vi "Actor Core.vi"(8 "error in":errorcluster, 11 "PLC_Module in":refnum<class "PLC_Module.lvclass">) -> (0 "error out":errorcluster, 3 "Actor out":refnum<class "Actor.lvclass">)   [LabVIEW 2025, in "PLC_Module.lvlib" / "PLC_Module.lvclass"]
doc: "<p>(<strong>Filename</strong>: <span class=\"dnl\">Actor Framework.lvlib:Actor.lvclass:Actor Core.vi</span>)</p>\n<p>Receives messages to the actor, reacts to them, and initiates any error handling that may shut the actor down.</p>\n<p>Descendant classes may override this VI to append parallel tasks for the actor to complete while it handles messages. Overrides use the <a href=\"nihelplauncher://docs/csh?context=lvcore_glang_udclass\">Call Parent Class Method</a> node.</p>"
uses:
  PLC_Module.lvclass
  <vilib>/ActorFramework/Actor/Actor.lvclass
  Msg&Data.ctl
  Msg.ctl
  PLC_Module.lvclass/PLC_Module.ctl
  <vilib>/ActorFramework/Actor/Actor.lvclass/Actor.ctl
  <vilib>/ActorFramework/Message Enqueuer/Message Enqueuer.lvclass/Message Enqueuer.ctl
  PLC_Module Messages/Rename Msg/Rename Msg.lvclass/Rename Msg.ctl
  PLC_Module Messages/Set Data Msg/Set Data Msg.lvclass/Set Data Msg.ctl
  PLC_Module Messages/Write Monitor Msg/Write Monitor Msg.lvclass/Write Monitor Msg.ctl
  UI_Object.ctl
  PLC_Module Messages/UI_Initialize Msg/UI_Initialize Msg.lvclass/UI_Initialize Msg.ctl
  PLC_Module Messages/Connection Msg/Connection Msg.lvclass/Connection Msg.ctl
  PLC_Module Messages/EditPanel Msg/EditPanel Msg.lvclass/EditPanel Msg.ctl
  <vilib>/addons/_JKI Toolkits/State Machine/_JKI_lib_State_Machine.llb/Select State(s)_err__jki_lib_state_machine.vi
  Read Configuration.vi
  Read ModuleName.vi
  Read ConnectConfig.vi
  Write ConnectConfig.vi
  <vilib>/ActorFramework/Message Enqueuer/Init from Existing Queue.vi
  <vilib>/ActorFramework/Message Enqueuer/Enqueue.vi
  PLC_Module Messages/PanelClose Msg/PanelClose Msg.lvclass
  PLC_Module Messages/Rename Msg/Rename Msg.lvclass
  PLC_Module Messages/Set Data Msg/Set Data Msg.lvclass
  PLC_Module Messages/Write Monitor Msg/Write Monitor Msg.lvclass
  <vilib>/ActorFramework/Stop Msg/Stop Msg.lvclass
  PLC_Module Messages/UI_Initialize Msg/UI_Initialize Msg.lvclass
  PLC_Module Messages/Monitor Msg/Monitor Msg.lvclass
  PLC_Module Messages/Connection Msg/Connection Msg.lvclass
  PLC_Module Messages/Disconnection Msg/Disconnection Msg.lvclass
  PLC_Module Messages/EditPanel Msg/EditPanel Msg.lvclass
  PLC_Module Messages/Delete Item Msg/Delete Item Msg.lvclass
  PLC_Module Messages/DuplicateItem Msg/DuplicateItem Msg.lvclass
  <vilib>/addons/_JKI Toolkits/State Machine/_JKI_lib_State_Machine.llb/Periodic Trigger__ogtk__JKI-SM__jki_lib_state_machine.vi
  <vilib>/ActorFramework/Message Priority Queue/Priority Enqueue.vi
  <vilib>/ActorFramework/Message Enqueuer/Message Enqueuer.lvclass
panel:
  in  "Listbox":i32[](listbox)
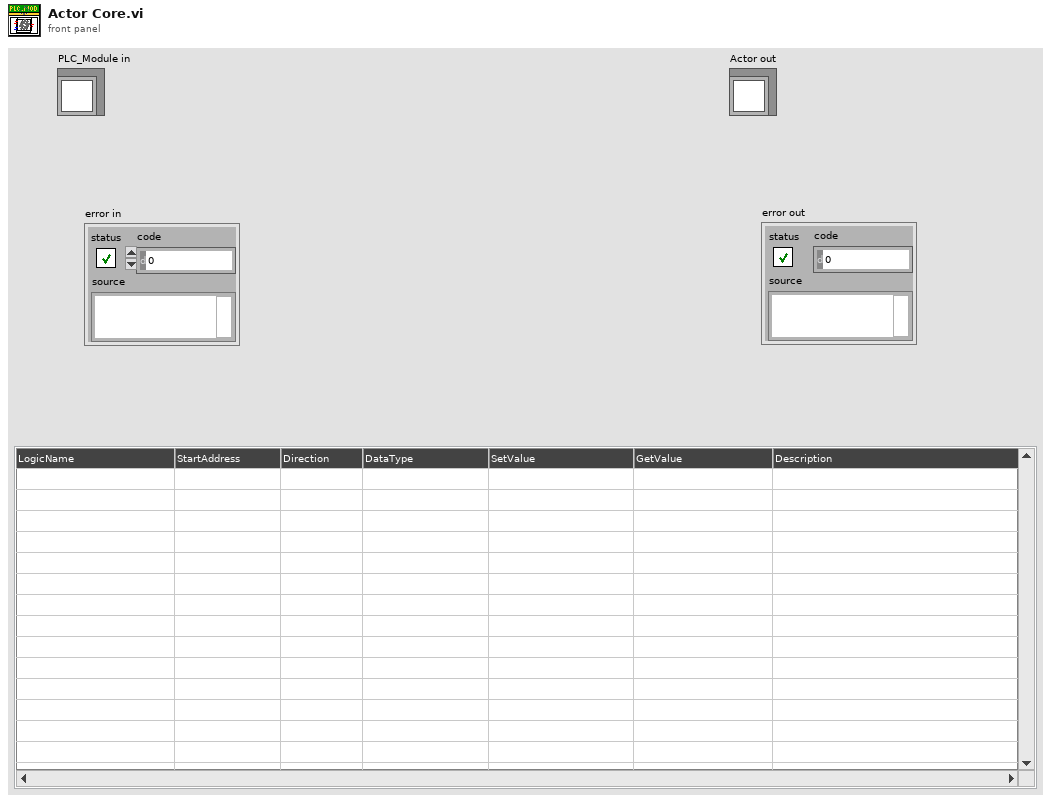
[diagram p1: front panel]
types:
  T1 = typedef "Msg&Data.ctl" = cluster{"Msg":T2, "Data":variant}
  T2 = typedef "Msg.ctl" = string
  T3 = enum32{"Invalid", "Standard", "Closed", "Hidden", "Minimized", "Maximized"}
  T4 = enum32{"invalid app kind", "Development System", "Run Time System", "Student Edition", "Embedded LabVIEW", "Evaluation", "Custom"}
  T5 = typedef "PLC_Module.lvlib/PLC_Module.lvclass/UI_Object.ctl" = cluster{"Core":cluster{"Current VI Reference":refnum<vi>, "Close Panel on Exit?":bool}, "Listbox":refnum<vi>}
  T6 = typedef "LVPoint32TypeDef.ctl" = cluster{"Horizontal":i32, "Vertical":i32}
  T7 = typedef "LVRowAndColumnTypeDef.ctl" = cluster{"Row":i32, "Column":i32}
  T8 = cluster{"Current VI Reference":refnum<vi>, "Close Panel on Exit?":bool}
  T9 = typedef "PLC_Module.lvlib/PLC_Module.lvclass/PLC_Data_Config.ctl" = map{string, cluster{"Config":T10, "Get Value":string, "Set Value":string}}
  T10 = typedef "PLC_Module.lvlib/PLC_Module.lvclass/PLC_Data.ctl" = cluster{"Address":string, "Direction":enum16{"PC->PLC", "PLC->PC"}, "DataType":T11, "Description":string}
  T11 = typedef "PLC_Module.lvlib/PLC_Module.lvclass/PLC_Data_Type.ctl" = enum16{"Boolean", "Single Float", "U8", "U32", "U32_Array", "String"}
  T12 = typedef "PLC_Module.lvlib/PLC_Module.lvclass/PLC_Connect_Config.ctl" = cluster{"IP Address":string, "Port":u16, "Timeout":i32}
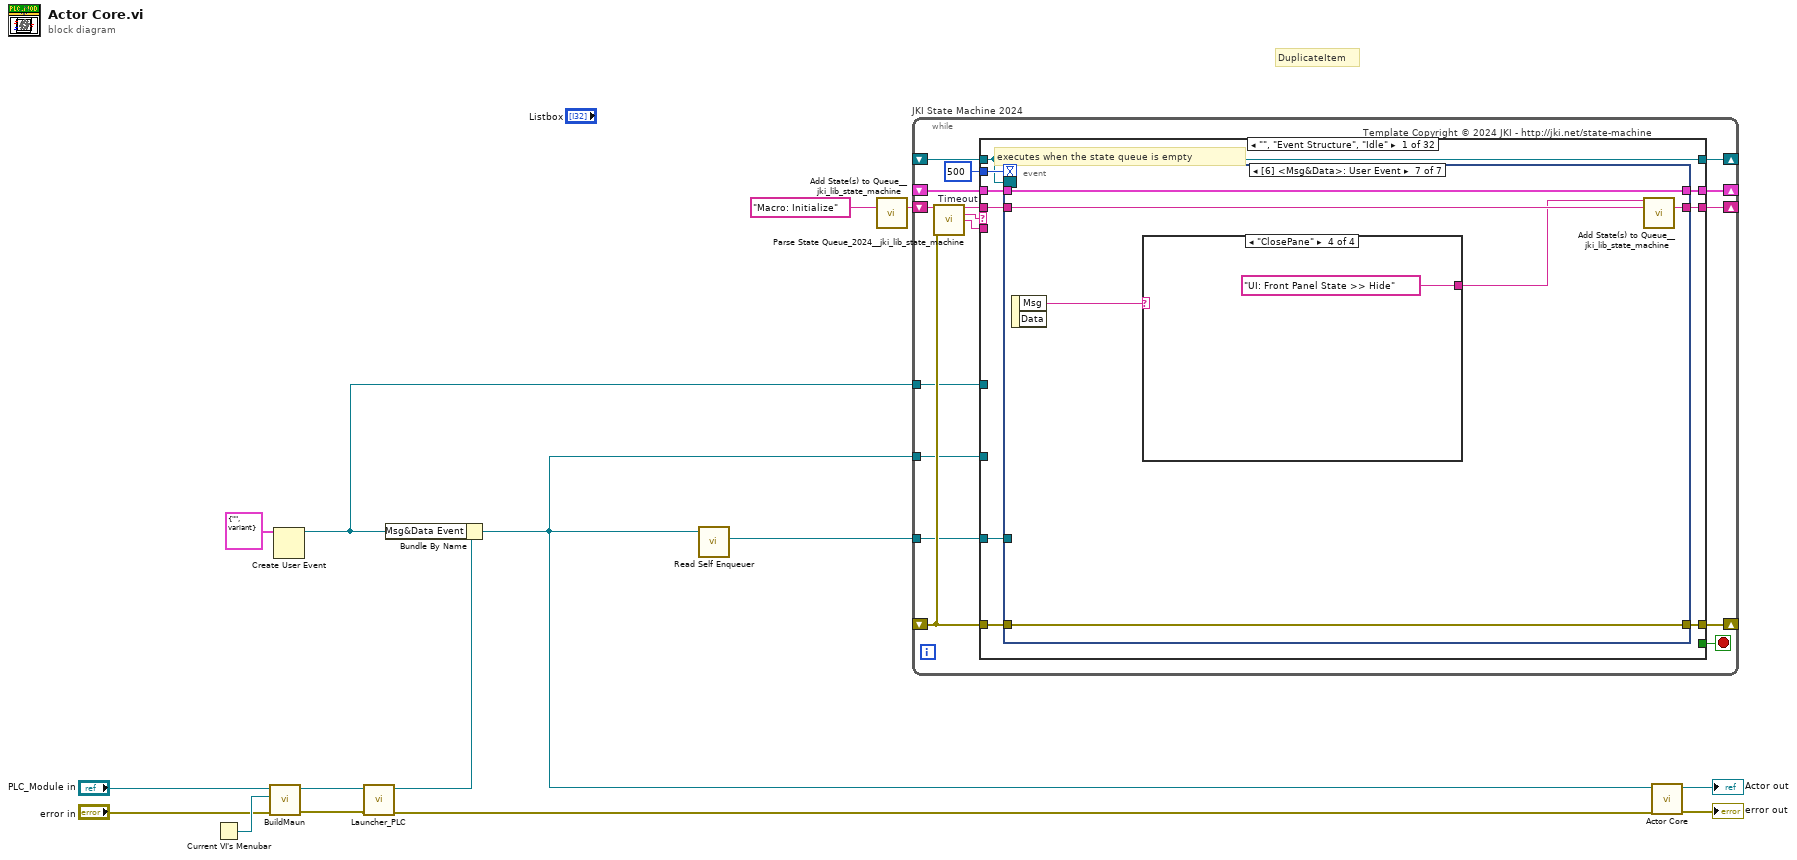
[diagram p0: block diagram]
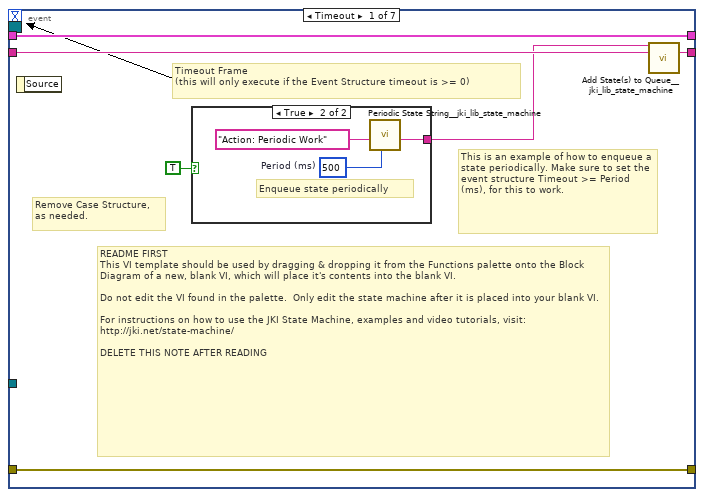
[diagram p2: hidden frame]
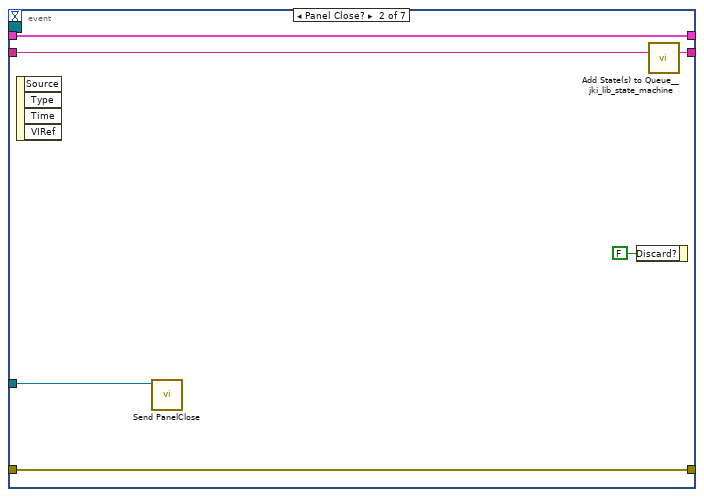
[diagram p4: hidden frame]
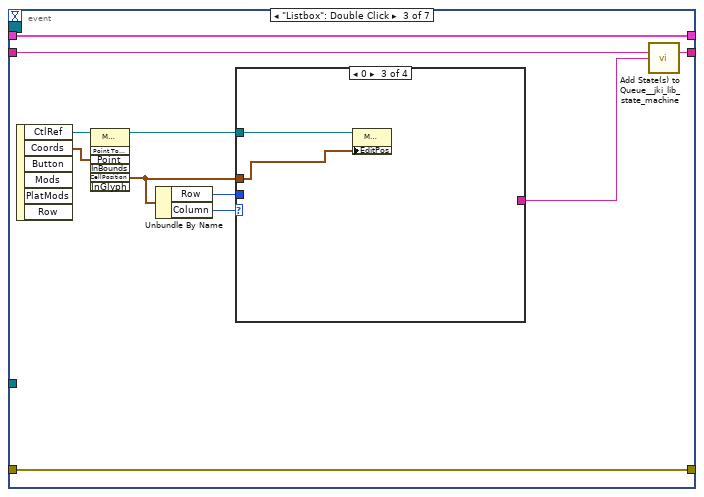
[diagram p5: hidden frame]
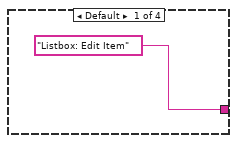
[diagram p6: hidden frame]
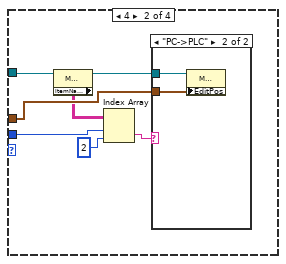
[diagram p7: hidden frame]
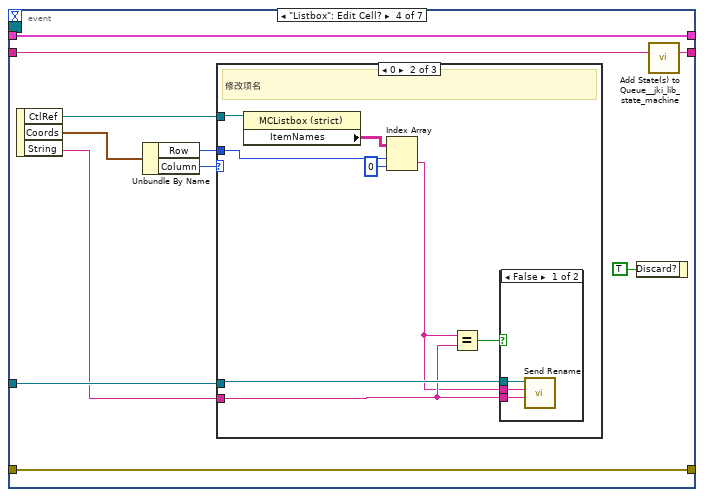
[diagram p10: hidden frame]
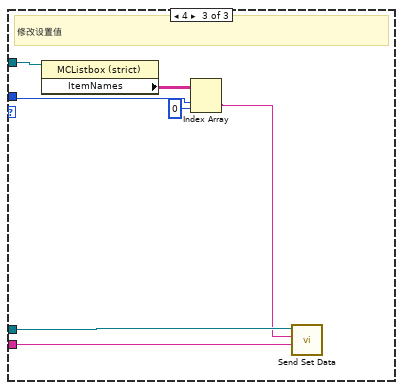
[diagram p13: hidden frame]
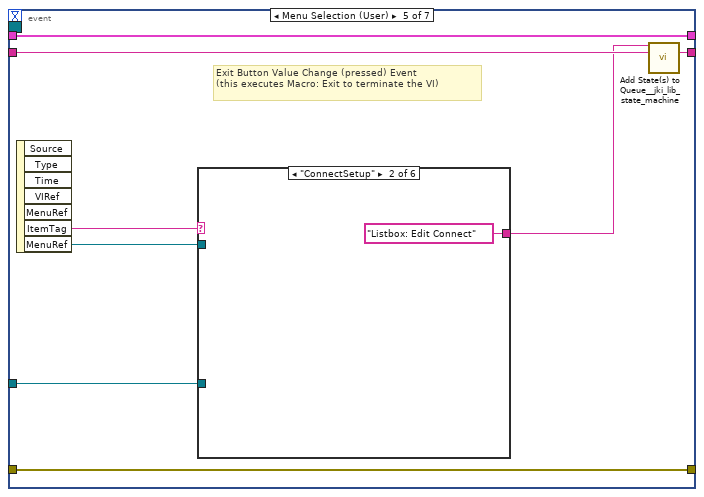
[diagram p14: hidden frame]
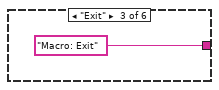
[diagram p16: hidden frame]
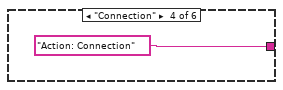
[diagram p17: hidden frame]
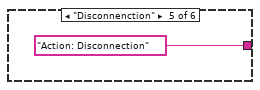
[diagram p18: hidden frame]
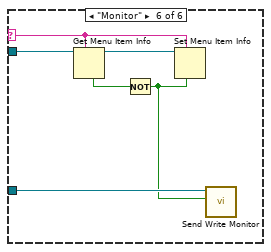
[diagram p19: hidden frame]
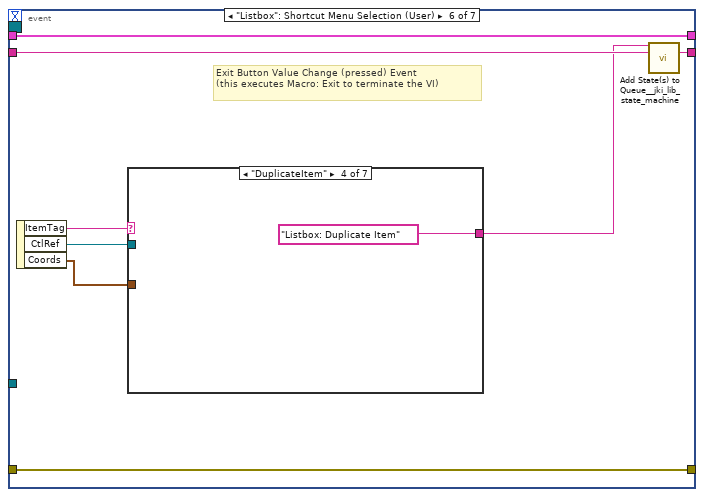
[diagram p20: hidden frame]
diagram:
  # "DuplicateItem"
  n1 = Current VI's Menubar() -> (w8:refnum<k9>)
  n2 = call "BuildMaun.vi"("error in (no error)"="error in", "menu reference"=w8, "PLC_Module in"="PLC_Module in") -> ("error out"=w3:errorcluster, "PLC_Module out"=w5:refnum<class "PLC_Module.lvclass">)  [unwired: 7 in]
  n3 = Create User Event(user event datatype=T1 {"Msg"="", "Data"=variant} ("Msg&Data")) -> (user event=w9:refnum<user-event>)  [unwired: 1 in, 1 out]
  n4 = call "Launcher_PLC.vi"("error in (no error)"=w3, "PLC_Module in"=w5) -> ("error out"=w2:errorcluster, "PLC_Module out"=w4:refnum<class "PLC_Module.lvclass">)  [unwired: 8 in]
  n5 = Bundle By Name(cluster=w4, "Msg&Data Event"=w9) -> (w1:refnum<class "PLC_Module.lvclass">)
  n6 = call <vilib>:"Read Self Enqueuer.vi"("Actor"=w1) -> ("Self Enqueuer"=w11:refnum<class "Message Enqueuer.lvclass">)  [unwired: 10 in]
  n7 = call <vilib>:"Add State(s) to Queue__jki_lib_state_machine.vi"("State(s) in (\"\")"="Macro: Initialize") -> ("States Out"=w13:string)  [unwired: 14 in]
  n8 = while "JKI State Machine 2024" {
    shift-right: [w24] -> _
    shift-left: _ -> [w23]
    shift-right: [w27] -> _
    shift-left: _ -> [w21]
    shift-right: [w26] -> _
    shift-left: w13 -> [w28]
    tunnel: w11 -> [w20]
    shift-right: [w19] -> _
    shift-left: _ -> [w18]
    tunnel: w9 -> [w17]
    tunnel: w1 -> [w16]
    stop <- w25 stop-if-true
    w22 = 500  # Timeout
    # "Template Copyright © 2024 JKI - http://jki.net/state-machine"
    n9 = call <vilib>:"Parse State Queue_2024__jki_lib_state_machine.vi"("State Queue"=w28, "Error In (no error)"=w21) -> ("Remaining States"=w30:string, "Current State"=w31:string, "Arguments"=w29:string)  [unwired: 11 in]
    n10 = case shown="\"\", \"Event Structure\", \"Idle\"" w31 {
      selector: w31 -> [_ _ w162 _ _ _ _ _ _ _ _ _ _ _ _ _ _ _ _ _ _ _ _ _ _ _ _ _ _ _ _ _]
      tunnel: w30 -> [w40 w160 w166 w186 w197 w209 w214 w222 w229 w234 w241 w247 w252 w260 w265 w272 w284 w354 w360 w370 w375 w381 w387 w393 w398 w405 w412 w417 w426 w432 w441 w447]
      tunnel: w29 -> [_ _ _ _ w192 _ _ _ _ _ _ _ _ _ _ w267 w278 _ _ _ _ _ _ _ _ _ _ _ _ _ _ _]
      tunnel: w23 -> [w38 w157 w164 w179 w194 w207 w211 _ w224 w231 w239 w245 w249 w255 w263 w270 w280 w351 w357 w368 w372 w378 w384 w390 w395 w402 w409 w414 w423 w429 w438 w444]
      tunnel: [w37 w158 w168 w183 errorcluster {"status"=FALSE, "code"=0, "source"=""} ("error out") w202 w212 w219 w225 w232 w237 w242 w250 w258 w262 w268 w281 w352 w358 w365 w373 w379 w385 w391 w396 w403 w410 w415 w424 w430 w439 w445] -> w27
      tunnel: w21 -> [w34 w158 w167 w183 w193 w203 w212 w219 w226 w232 w236 w243 w250 w258 w262 w269 w282 w352 w358 w365 w373 w379 w385 w391 w396 w403 w410 w415 w424 w430 w439 w445]
      tunnel: [w39 w159 w165 w185 w196 w208 w213 w221 w228 w233 w240 w246 w251 w259 w264 w271 w283 w353 w359 w369 w374 w380 w386 w392 w397 w404 w411 w416 w425 w431 w440 w446] -> w26
      tunnel: [_ _ _ _ _ TRUE _ _ _ _ _ _ _ _ _ _ _ _ _ _ _ _ _ _ _ _ _ _ _ _ _ _] -> w25
      tunnel: [w36 w157 w164 w184 w194 w207 w211 w220 w224 w231 w239 w245 w249 w255 w263 w270 w280 w351 w357 w368 w372 w378 w384 w390 w395 w402 w409 w414 w423 w429 w438 w444] -> w24
      tunnel: w22 -> [w35 _ _ _ _ _ _ _ _ _ _ _ _ _ _ _ _ _ _ _ _ _ _ _ _ _ _ _ _ _ _ _]
      tunnel: w20 -> [w32 _ _ _ _ w204 _ _ _ _ _ _ _ w256 _ _ _ _ _ _ _ w376 w382 w388 _ w399 w407 _ _ w427 _ w442]
      tunnel: [w33 w156 w161 w173 w187 w205 w210 w217 w223 w230 w238 w244 w248 w257 w261 w266 w277 w350 w355 w361 w371 w377 w383 w389 w394 w401 w408 w413 w422 w428 w437 w443] -> w19
      tunnel: w18 -> [w33 w156 w161 w173 w187 w205 w210 w217 w223 w230 _ w244 w248 w257 w261 w266 w277 w350 w355 w361 w371 w377 w383 w389 w394 w401 w408 w413 w422 w428 w437 w443]
      tunnel: w17 -> [_ _ _ _ _ _ _ _ _ _ w235 _ _ _ _ _ _ _ _ _ _ _ _ _ _ _ _ _ _ _ _ _]
      tunnel: w16 -> [_ _ _ _ _ _ _ _ _ _ _ _ _ _ _ _ _ _ _ _ _ _ _ _ _ _ _ _ w421 _ w436 _]
      frame "", "Event Structure", "Idle" {
        # "executes when the state queue is empty"
        n11 = event shown="[6] <Msg&Data>: User Event" {
          selector: w33 -> [_ _ _ _ _ _ _]
          dyn-events: _ -> [_ _ _ _ _ _ _]
          timeout: w35 -> [_ _ _ _ _ _ _]
          tunnel: w40 -> [w46 w55 w66 w89 w115 w133 w152]
          tunnel: [w45 w54 w65 w88 w114 w132 w151] -> w39
          tunnel: w38 -> [w43 w52 w63 w86 w112 w130 w149]
          tunnel: [w44 w53 w64 w87 w113 w131 w150] -> w37
          tunnel: w34 -> [w44 w53 w64 w87 w113 w131 w150]
          tunnel: [w43 w52 w63 w86 w112 w130 w149] -> w36
          tunnel: w32 -> [_ w50 _ w84 w108 _ _]
          event Timeout {
            # "Remove Case Structure, as needed."
            # "This is an example of how to enqueue a state periodically. Make sure to set the event structure Timeout >= Period (ms), for this to work."
            # "README FIRST\nThis VI template should be used by dragging & dropping it from the Functions palette onto the Block Diagram of a new, blank VI, which will place it's contents into the blank VI.\n\nDo not edit the VI found in the palette.  Only edit the state machine after it is placed into your blank VI.\n\nFor instructions on how to use the JKI State Machine, examples and video tutorials, visit:\nhttp://jki.net/state-machine/\n\nDELETE THIS NOTE AFTER READING"
            # "Timeout Frame\n(this will only execute if the Event Structure timeout is >= 0)"
            n12 = event-data() -> ()  [unwired: 1 in, 1 out]
            n13 = case shown="True" TRUE {
              tunnel: [_ w49] -> w42
              frame False {
              }
              frame True {
                w47 = u32 500  # Period (ms)
                # "Enqueue state periodically"
                n14 = call <vilib>:"Periodic State String__jki_lib_state_machine.vi"("Period (ms)"=w47, "State"="Action: Periodic Work") -> ("State Out"=w49:string)  [unwired: 9 in]
              }
            }
            n15 = call <vilib>:"Add State(s) to Queue__jki_lib_state_machine.vi"("State(s) in Front (\"\")"=w42, "State(s) in (\"\")"=w46) -> ("States Out"=w45:string)  [unwired: 13 in]
          }
          event Panel Close? {
            n16 = event-data() -> ()  [unwired: 1 in, 4 out]
            n17 = call "Send PanelClose.vi"("Message Enqueuer"=w50) -> ()  [unwired: 9 in, 2 out]
            n18 = event-data("Discard?"=FALSE) -> ()  [unwired: 1 in, 1 out]
            n19 = call <vilib>:"Add State(s) to Queue__jki_lib_state_machine.vi"("State(s) in (\"\")"=w55) -> ("States Out"=w54:string)  [unwired: 14 in]
          }
          event "Listbox": Double Click {
            n20 = event-data() -> ("CtlRef"=w62:refnum<vi>, "Coords"=w61:T6)  [unwired: 1 in, 4 out]
            n21 = invoke class="MCListbox (strict)" method="Point To Row Column"(reference=w62, "Point"=w61) -> (reference out=w58:refnum<vi>, "CellPosition"=w57:T7)  [unwired: 5 in, 5 out]
            n22 = Unbundle By Name(w57) -> ("Row"=w56:i32, "Column"=w60:i32)
            n23 = case shown="0" w60 {
              tunnel: ["Listbox: Edit Item" _ _ _] -> w59
              tunnel: w58 -> [_ w74 w78 _]
              tunnel: w57 -> [_ w73 w77 _]
              tunnel: w56 -> [_ w70 _ _]
              frame Default {
              }
              frame 4 {
                n24 = property class="MCListbox (strict)"(reference=w74) -> (reference out=w72:refnum<vi>, "ItemNames"=w71:string[][])  [unwired: 1 in, 1 out]
                n25 = Index Array(array=w71, index (row)=w70, index (col)=2 ("disabled index (col)")) -> (element=w68:string)
                n26 = case shown="\"PC->PLC\"" w68 {
                  tunnel: w73 -> [_ w76]
                  tunnel: w72 -> [_ w75]
                  frame Default {
                  }
                  frame "PC->PLC" {
                    n27 = property class="MCListbox (strict)"(reference=w75, "EditPos"=w76) -> ()  [unwired: 1 in, 2 out]
                  }
                }
              }
              frame 0 {
                n28 = property class="MCListbox (strict)"(reference=w78, "EditPos"=w77) -> ()  [unwired: 1 in, 2 out]
              }
              frame 5 {
              }
            }
            n29 = call <vilib>:"Add State(s) to Queue__jki_lib_state_machine.vi"("State(s) in (\"\")"=w66, "State(s) at Back (\"\")"=w59) -> ("States Out"=w65:string)  [unwired: 13 in]
          }
          event "Listbox": Edit Cell? {
            n30 = event-data() -> ("CtlRef"=w82:refnum<vi>, "Coords"=w81:T7, "String"=w83:string)  [unwired: 1 in]
            n31 = Unbundle By Name(w81) -> ("Row"=w80:i32, "Column"=w79:i32)
            n32 = case shown="0" w79 {
              tunnel: w84 -> [_ w97 w107]
              tunnel: w83 -> [_ w92 w106]
              tunnel: w82 -> [_ w96 w102]
              tunnel: w80 -> [_ w94 w101]
              frame Default {
              }
              frame 0 {
                # "修改项名"
                n33 = property class="MCListbox (strict)"(reference=w96) -> ("ItemNames"=w95:string[][])  [unwired: 1 in, 2 out]
                n34 = Index Array(array=w95, index (row)=w94, index (col)=0 ("disabled index (col)")) -> (element=w91:string)
                n35 = Equal?(x=w91, y=w92) -> (x = y?=w90:bool)
                n36 = case shown="False" w90 {
                  tunnel: w97 -> [w100 _]
                  tunnel: w92 -> [w99 _]
                  tunnel: w91 -> [w98 _]
                  frame False {
                    n37 = call "Send Rename.vi"("NewName"=w99, "OldName"=w98, "Message Enqueuer"=w100) -> ()  [unwired: 7 in, 2 out]
                  }
                  frame True {
                  }
                }
              }
              frame 4 {
                # "修改设置值"
                n38 = property class="MCListbox (strict)"(reference=w102) -> ("ItemNames"=w105:string[][])  [unwired: 1 in, 2 out]
                n39 = Index Array(array=w105, index (row)=w101, index (col)=0 ("disabled index (col)")) -> (element=w103:string)
                n40 = call "Send Set Data.vi"("Set Value"=w106, "LogicName"=w103, "Message Enqueuer"=w107) -> ()  [unwired: 7 in, 2 out]
              }
            }
            n41 = event-data("Discard?"=TRUE) -> ()  [unwired: 1 in, 1 out]
            n42 = call <vilib>:"Add State(s) to Queue__jki_lib_state_machine.vi"("State(s) in (\"\")"=w89) -> ("States Out"=w88:string)  [unwired: 14 in]
          }
          event Menu Selection (User) {
            # "Exit Button Value Change (pressed) Event\n(this executes Macro: Exit to terminate the VI)"
            n43 = event-data() -> ("ItemTag"=w111:string, "MenuRef"=w109:refnum<k9>)  [unwired: 1 in, 5 out]
            n44 = case shown="\"ConnectSetup\"" w111 {
              selector: w111 -> [_ _ _ _ _ w122]
              tunnel: [_ "Listbox: Edit Connect" "Macro: Exit" "Action: Connection" "Action: Disconnection" _] -> w110
              tunnel: w109 -> [_ _ _ _ _ w125]
              tunnel: w108 -> [_ _ _ _ _ w121]
              frame Default {
              }
              frame "ConnectSetup" {
              }
              frame "Exit" {
              }
              frame "Connection" {
              }
              frame "Disconnenction" {
              }
              frame "Monitor" {
                n45 = Get Menu Item Info(7:w122, 11:w125) -> (3:w124:refnum<k9>, 4:w123:bool)  [unwired: 1 in, 5 out]
                n46 = Not(x=w123) -> (.not. x?=w120:bool)
                n47 = Set Menu Item Info(6:w120, 7:w122, 11:w124) -> ()  [unwired: 4 in, 2 out]
                n48 = call "Send Write Monitor.vi"("Monitor"=w120, "Message Enqueuer"=w121) -> ()  [unwired: 8 in, 2 out]
              }
            }
            n49 = call <vilib>:"Add State(s) to Queue__jki_lib_state_machine.vi"("State(s) in Front (\"\")"=w110, "State(s) in (\"\")"=w115) -> ("States Out"=w114:string)  [unwired: 13 in]
          }
          event "Listbox": Shortcut Menu Selection (User) {
            # "Exit Button Value Change (pressed) Event\n(this executes Macro: Exit to terminate the VI)"
            n50 = event-data() -> ("ItemTag"=w129:string, "CtlRef"=w127:refnum<vi>, "Coords"=w126:T6)  [unwired: 1 in]
            n51 = case shown="\"DuplicateItem\"" w129 {
              tunnel: [_ _ "Listbox: Add Item" "Listbox: Duplicate Item" "Listbox: Edit Item" "Listbox: Delete Item" "Listbox: Save Config"] -> w128
              tunnel: w127 -> [_ w141 _ _ _ _ _]
              tunnel: w126 -> [_ w140 _ _ _ _ _]
              frame Default {
              }
              frame "CopyLogicName" {
                n52 = invoke class="MCListbox (strict)" method="Point To Row Column"(reference=w141, "Point"=w140) -> (reference out=w139:refnum<vi>, "CellPosition"=w137:T7)  [unwired: 5 in, 5 out]
                n53 = property class="MCListbox (strict)"(reference=w139) -> ("ItemNames"=w138:string[][])  [unwired: 1 in, 2 out]
                n54 = Unbundle(w137) -> ("Row"=w136:i32)  [unwired: 1 out]
                n55 = Index Array(array=w138, index (row)=w136, index (col)=0 ("disabled index (col)")) -> (element=w134:string)
                n56 = invoke class="App" method="Clipboard.Write"("Param 0"=w134) -> ()  [unwired: 3 in, 4 out]
              }
              frame "AddItem" {
              }
              frame "DuplicateItem" {
              }
              frame "EditItem" {
              }
              frame "DeleteItem" {
              }
              frame "SaveConfig" {
              }
            }
            n57 = call <vilib>:"Add State(s) to Queue__jki_lib_state_machine.vi"("State(s) in Front (\"\")"=w128, "State(s) in (\"\")"=w133) -> ("States Out"=w132:string)  [unwired: 13 in]
          }
          event User Event {
            n58 = event-data() -> ("Msg"=w148:T2)  [unwired: 1 in, 1 out]
            n59 = case shown="\"ClosePane\"" w148 {
              tunnel: [_ "Macro: Exit" "UI: Front Panel State >>Open" "UI: Front Panel State >> Hide"] -> w147
              frame Default {
              }
              frame "Exit" {
              }
              frame "OpenPane" {
              }
              frame "ClosePane" {
              }
            }
            n60 = call <vilib>:"Add State(s) to Queue__jki_lib_state_machine.vi"("State(s) in Front (\"\")"=w147, "State(s) in (\"\")"=w152) -> ("States Out"=w151:string)  [unwired: 13 in]
          }
        }
      }
      frame "---------- Core ----------" {
        # "Do not put any code in this frame.\n(it is a separator no-op)"
        n61 = call <vilib>:"Add State(s) to Queue__jki_lib_state_machine.vi"("State(s) in (\"\")"=w160) -> ("States Out"=w159:string)  [unwired: 14 in]
      }
      frame Default {
        w171 = 42 items=["No error", "Argument error", "Memory is full", "Out of zone", "End of file", "File already open", "Generic file I/O error", "File not found", "File permission error", "Disk is full", "Duplicate path", "Too many files open", "System feature not enabled", "Resource file not found", "Cannot add resource", "Resource not found", "Image not found", "Image memory error", "Pen does not exist", "Config type invalid", "Config token not found", "Config parse error", "Config memory error", "Bad external code format", "Bad external code offset", "External code not present", "Null window", "Destroy window error", "Null menu", "Print aborted", "Bad print record", "Print driver error", "Windows error during printing", "Memory error during printing", "Print dialog error", "Generic print error", "Invalid device refnum", "Device not found", "Device parameter error", "Device unit error", "Cannot open device", "Device call aborted", "Generic error", "Cancelled by user", "Object ID too low", "Object ID too high", "Object not in heap", "Unknown heap", "Unknown object (invalid DefProc)", "Unknown object (DefProc not in table)", "Message out of range", "Invalid (null) method", "Unknown message", "Manager call not supported", "Bad address", "Network operation in progress", "Network operation timed out", "Connection is busy", "Network attribute not supported", "Network error", "Address in use", "System out of memory", "Connection aborted", "Connection refused", "Not connected", "Already connected", "Connection closed", "Initialization error (interapplication manager)", "Bad occurrence", "Wait on unbound occurrence handler", "Occurrence queue overflow", "Datalog type conflict", "Unused", "Unrecognized type (interapplication manager)", "Memory corrupt", "Failed to make temporary DLL", "Old CIN version", "Drag socket not found", "Failed to load drop-object", "Failed to register OLE object", "Failed to release OLE object", "Format specifier type mismatch", "Unknown format specifier", "Too few format specifiers", "Too many format specifiers", "Scan failed", "Newer CIN version", "Error converting to variant", "Runtime menu error", "Password tampered", "Variant attribute not found", "Incompatible variant data type", "Event data is not available", "Event Store is not present", "Occurrence is not found", "Event Queue is not created", "Event info is not available", "Refnum passed is NULL", "Error retrieving Class GUID", "Error retrieving CoClass GUID", "Error retrieving TypeLib GUID.", "Bad built application magic bytes.", "Specific driver is different from the specific driver associated with the Logical Name.", "There is no session opened to the class driver.", "Max Error", "MAX - Error with config objects", "MAX - Error loading configuration", "MAX - Group not supported"]
        # "Current State"
        # "Do not delete, rename, or modify this frame.\n(this is used to capture unhandled states and typos)"
        # "Handle mistyped state name (developer tool)"
        n62 = Format Into String(format string="Software Exception: Unhandled State \"%s\"." ("message"), error in=w167, w162) -> (resulting string=w170:string, error out=w169:errorcluster)  [unwired: 1 in]
        n63 = call <vilib>:"Error Cluster From Error Code.vi"("show call chain? (False)"=TRUE, "error in (no error)"=w169, "error message (\"\")"=w170, "error code (0)"=w171) -> ("error out"=w168:errorcluster)  [unwired: 5 in]
        n64 = call <vilib>:"Add State(s) to Queue__jki_lib_state_machine.vi"("State(s) in (\"\")"=w166) -> ("States Out"=w165:string)  [unwired: 14 in]
      }
      frame "Initialize Core Data" {
        # "Do not delete, rename, or modify this frame.\n(this is used to determine panel behavior on exit)"
        # "originally closed?"
        # "exe?"
        # "If panel starts closed or is an EXE, then close it when we exit"
        n65 = property class="VI"() -> ("FP.State"=w176:T3)  [unwired: 2 in, 2 out]
        n66 = property class="App"() -> ("App.Kind"=w182:T4)  [unwired: 2 in, 2 out]
        n67 = control-ref of="Current VI Reference"() -> (w177:refnum<vi>)
        n68 = Equal?(x=w176, y=T3."Closed" ("Front Panel Window:State")) -> (x = y?=w174:bool)
        n69 = Equal?(x=w182, y=T4."Run Time System" ("Application:Kind")) -> (x = y?=w180:bool)
        n70 = Or(x=w174, y=w180) -> (x .or. y?=w178:bool)
        n71 = Bundle By Name(cluster=w179, "Core.Current VI Reference"=w177, "Core.Close Panel on Exit?"=w178) -> (w184:T5)
        n72 = call <vilib>:"Add State(s) to Queue__jki_lib_state_machine.vi"("State(s) in (\"\")"=w186) -> ("States Out"=w185:string)  [unwired: 14 in]
      }
      frame "Error Handler" {
        # "When running as sourcecode, this function will add previous state data to the error message to aid the developer in troubleshoot errors.\nIf run as an executable, no additional information is added to the error message."
        # "This state receives both Errors and Warnings which is how the Status of this wire can be FALSE"
        # "Unhandled Error -- Display it"
        # "Handle any errors or warnings here.\nYou can also output any states to clean-up after errors or warnings occur"
        # "Clear error or warning"
        n73 = disable-structure shown="Default" {
          disable-tunnel: w193 -> [w200 w201]
          disable-tunnel: w192 -> [w199 _]
          disable-tunnel: [w198 w201] -> w191
          frame condition #0 (active) {
            n74 = call <vilib>:"Append Error Details__jki_lib_state_machine.vi"("error in (no error)"=w200, "Previous State and Argument(s)"=w199) -> ("error out"=w198:errorcluster)  [unwired: 9 in]
          }
          frame condition #1 {
          }
        }
        n75 = call <vilib>:"General Error Handler.vi"("error in (no error)"=w191) -> ()  [unwired: 10 in, 5 out]
        n76 = call-poly <vilib>:"Select State(s)__jki_lib_state_machine.vi"("State(s) if True (\"\")"="/* Post Error States", "Select"=w191, "State(s) if False (\"\")"="/* Post Warning States") -> ("States Out"=w189:string)  [unwired: 12 in]
        n77 = call <vilib>:"Add State(s) to Queue__jki_lib_state_machine.vi"("State(s) in Front (\"\")"=w189, "State(s) in (\"\")"=w197) -> ("States Out"=w196:string)  [unwired: 13 in]
      }
      frame "Exit" {
        # "Do not put any code in this frame.\n(No errors that occur here will be handled.)"
        n78 = call <vilib>:"Send Normal Stop.vi"("error in (no error)"=w203, "Message Enqueuer"=w204) -> ("error out"=w202:errorcluster)  [unwired: 9 in]
        n79 = call <vilib>:"Add State(s) to Queue__jki_lib_state_machine.vi"("State(s) in (\"\")"=w209) -> ("States Out"=w208:string)  [unwired: 14 in]
      }
      frame "---------- Data ----------" {
        # "Do not put any code in this frame.\n(It is a separator no-op. You can make a copy of this frame to create a new Data frame)"
        n80 = call <vilib>:"Add State(s) to Queue__jki_lib_state_machine.vi"("State(s) in (\"\")"=w214) -> ("States Out"=w213:string)  [unwired: 14 in]
      }
      frame "Data: Initialize" {
        w218 = T8 {"Current VI Reference"=refnum, "Close Panel on Exit?"=FALSE}  # Core
        # "Data names and types of shift register data are defined by this bundle."
        # "Initialize the shift-register data, here.\n(data names are defined by what you wire into the bundle function)"
        n81 = control-ref of="Listbox"() -> (w216:refnum<vi>)
        n82 = Bundle(cluster=T5 {"Core"={"Current VI Reference"=refnum, "Close Panel on Exit?"=FALSE}, "Listbox"=refnum}, "Core"=w218, "Listbox"=w216) -> (w220:T5)
        n83 = call <vilib>:"Add State(s) to Queue__jki_lib_state_machine.vi"("State(s) in (\"\")"=w222) -> ("States Out"=w221:string)  [unwired: 14 in]
      }
      frame "Data: Cleanup" {
        # "Cleanup any data and references, here.\n(this is called automatically, by the Macro: Exit)"
        n84 = Unbundle By Name(w224) -> ("Core.Current VI Reference"=w227:refnum<vi>)
        n85 = Close Reference(reference=w227, error in (no error)=w226) -> (error out=w225:errorcluster)
        n86 = call <vilib>:"Add State(s) to Queue__jki_lib_state_machine.vi"("State(s) in (\"\")"=w229) -> ("States Out"=w228:string)  [unwired: 14 in]
      }
      frame "---------- Events ----------" {
        # "Do not put any code in this frame.\n(It is a separator no-op. You can make a copy of this frame to create a new UI frame)"
        n87 = call <vilib>:"Add State(s) to Queue__jki_lib_state_machine.vi"("State(s) in (\"\")"=w234) -> ("States Out"=w233:string)  [unwired: 14 in]
      }
      frame "Events: Register" {
        # "Do not put any code in this frame.\n(It is a separator no-op. You can make a copy of this frame to create a new UI frame)"
        n88 = register-events(error in=w236, w235) -> (reference out=w238:refnum<event-registration>, error out=w237:errorcluster)  [unwired: 1 in]
        n89 = call <vilib>:"Add State(s) to Queue__jki_lib_state_machine.vi"("State(s) in (\"\")"=w241) -> ("States Out"=w240:string)  [unwired: 14 in]
      }
      frame "Events: Unregister" {
        # "Do not put any code in this frame.\n(It is a separator no-op. You can make a copy of this frame to create a new UI frame)"
        n90 = Unregister For Events(event registration refnum=w244, error in=w243) -> (error out=w242:errorcluster)
        n91 = call <vilib>:"Add State(s) to Queue__jki_lib_state_machine.vi"("State(s) in (\"\")"=w247) -> ("States Out"=w246:string)  [unwired: 14 in]
      }
      frame "---------- UI ----------" {
        # "Do not put any code in this frame.\n(It is a separator no-op. You can make a copy of this frame to create a new UI frame)"
        n92 = call <vilib>:"Add State(s) to Queue__jki_lib_state_machine.vi"("State(s) in (\"\")"=w252) -> ("States Out"=w251:string)  [unwired: 14 in]
      }
      frame "UI: Initialize" {
        # "Initialize the User Interface, here.\n(this is called automatically, by the Macro: Initialize)"
        n93 = Unbundle By Name(w255) -> ("Listbox"=w254:refnum<vi>)
        n94 = property class="MCListbox (strict)"(reference=w254, "AlternatingRowColors"=TRUE ("Alternating Row Colors")) -> ()  [unwired: 1 in, 2 out]
        n95 = call "Send UI_Initialize.vi"("UI_Object"=w255, "Message Enqueuer"=w256) -> ()  [unwired: 8 in, 2 out]
        n96 = call <vilib>:"Add State(s) to Queue__jki_lib_state_machine.vi"("State(s) in (\"\")"=w260) -> ("States Out"=w259:string)  [unwired: 14 in]
      }
      frame "UI: Uninitialize" {
        # "Cleanup the User Interface, here.\n(this is called automatically, by the Macro: Exit)"
        n97 = call <vilib>:"Add State(s) to Queue__jki_lib_state_machine.vi"("State(s) in (\"\")"=w265) -> ("States Out"=w264:string)  [unwired: 14 in]
      }
      frame "UI: Cursor Set" {
        # "Argument"
        # "Set and Unset Cursor Busy.\n(Usage: \"UI: Cursor Set >> Busy|Idle\")"
        n98 = case shown="\"Idle\", Default" w267 {
          tunnel: w269 -> [w274 w276]
          tunnel: [w273 w275] -> w268
          frame "Idle", Default {
            n99 = call <vilib>:"Unset Busy.vi"("error in (no error)"=w274) -> ("error out"=w273:errorcluster)  [unwired: 10 in]
          }
          frame "Busy" {
            n100 = call <vilib>:"Set Busy.vi"("error in (no error)"=w276) -> ("error out"=w275:errorcluster)  [unwired: 9 in, 1 out]
          }
        }
        n101 = call <vilib>:"Add State(s) to Queue__jki_lib_state_machine.vi"("State(s) in (\"\")"=w272) -> ("States Out"=w271:string)  [unwired: 14 in]
      }
      frame "UI: Front Panel State" {
        # "Argument"
        # "Set Front Panel Open or Closed\n(Usage: \"UI: Front Panel State >> Open|Close\")"
        n102 = Unbundle By Name(w280) -> ("Core.Current VI Reference"=w279:refnum<vi>)
        n103 = case shown="\"Minimize\", \"Minimized\"" w278 {
          tunnel: w282 -> [w290 w305 w316 w329 w342]
          tunnel: [w292 w306 w318 w331 w344] -> w281
          tunnel: w279 -> [w291 w303 w317 w330 w343]
          frame "Open", "Standard", Default {
            w285 = T3."Standard" ("State")
            n104 = property class="VI"(reference=w291, error in=w290) -> (reference out=w288:refnum<vi>, error out=w289:errorcluster, "FP.State"=w287:T3)
            n105 = Not Equal?(x=w287, y=w285) -> (x != y?=w286:bool)
            n106 = case shown="True" w286 {
              tunnel: [w296 w298] -> w292
              tunnel: w289 -> [w295 w298]
              tunnel: w288 -> [w294 _]
              tunnel: w285 -> [w293 _]
              frame True {
                n107 = invoke class="VI" method="FP.Open"(reference=w294, error in=w295, "Activate"=TRUE, "State"=w293) -> (error out=w296:errorcluster)  [unwired: 1 in, 4 out]
              }
              frame False {
              }
            }
          }
          frame "Close", "Closed" {
            n108 = property class="VI"(reference=w303, error in=w305) -> (reference out=w302:refnum<vi>, error out=w304:errorcluster, "FP.State"=w300:T3)
            n109 = Not Equal?(x=w300, y=T3."Closed" ("Front Panel Window:State")) -> (x != y?=w299:bool)
            n110 = case shown="True" w299 {
              tunnel: [w307 w310] -> w306
              tunnel: w304 -> [w307 w309]
              tunnel: w302 -> [_ w308]
              frame False {
              }
              frame True {
                n111 = invoke class="VI" method="FP.Close"(reference=w308, error in=w309) -> (error out=w310:errorcluster)  [unwired: 1 in, 2 out]
              }
            }
          }
          frame "Hidden", "Hide" {
            w311 = T3."Hidden" ("State")
            n112 = property class="VI"(reference=w317, error in=w316) -> (reference out=w314:refnum<vi>, error out=w315:errorcluster, "FP.State"=w313:T3)
            n113 = Not Equal?(x=w313, y=w311) -> (x != y?=w312:bool)
            n114 = case shown="True" w312 {
              tunnel: [w322 w323] -> w318
              tunnel: w315 -> [w321 w323]
              tunnel: w314 -> [w320 _]
              tunnel: w311 -> [w319 _]
              frame True {
                n115 = invoke class="VI" method="FP.Open"(reference=w320, error in=w321, "State"=w319) -> (error out=w322:errorcluster)  [unwired: 2 in, 4 out]
              }
              frame False {
              }
            }
          }
          frame "Minimize", "Minimized" {
            w324 = T3."Minimized" ("State")
            n116 = property class="VI"(reference=w330, error in=w329) -> (reference out=w327:refnum<vi>, error out=w328:errorcluster, "FP.State"=w326:T3)
            n117 = Not Equal?(x=w326, y=w324) -> (x != y?=w325:bool)
            n118 = case shown="True" w325 {
              tunnel: [w335 w336] -> w331
              tunnel: w328 -> [w334 w336]
              tunnel: w327 -> [w333 _]
              tunnel: w324 -> [w332 _]
              frame True {
                n119 = invoke class="VI" method="FP.Open"(reference=w333, error in=w334, "State"=w332) -> (error out=w335:errorcluster)  [unwired: 2 in, 4 out]
              }
              frame False {
              }
            }
          }
          frame "Maximize", "Maximized" {
            w337 = T3."Maximized" ("State")
            n120 = property class="VI"(reference=w343, error in=w342) -> (reference out=w340:refnum<vi>, error out=w341:errorcluster, "FP.State"=w339:T3)
            n121 = Not Equal?(x=w339, y=w337) -> (x != y?=w338:bool)
            n122 = case shown="True" w338 {
              tunnel: [w348 w349] -> w344
              tunnel: w341 -> [w347 w349]
              tunnel: w340 -> [w346 _]
              tunnel: w337 -> [w345 _]
              frame True {
                n123 = invoke class="VI" method="FP.Open"(reference=w346, error in=w347, "State"=w345) -> (error out=w348:errorcluster)  [unwired: 2 in, 4 out]
              }
              frame False {
              }
            }
          }
        }
        n124 = call <vilib>:"Add State(s) to Queue__jki_lib_state_machine.vi"("State(s) in (\"\")"=w284) -> ("States Out"=w283:string)  [unwired: 14 in]
      }
      frame "---------- Macro ----------" {
        # "Do not put any code in this frame.\n(It is a separator no-op. You can make a copy of this frame to create a new Macro frame)"
        n125 = call <vilib>:"Add State(s) to Queue__jki_lib_state_machine.vi"("State(s) in (\"\")"=w354) -> ("States Out"=w353:string)  [unwired: 14 in]
      }
      frame "Macro: Initialize" {
        # "Initialization Macro\n(This is called once, when the VI starts)"
        n126 = call <vilib>:"Add State(s) to Queue__jki_lib_state_machine.vi"("State(s) in Front (\"\")"="Data: Initialize\nInitialize Core Data\nEvents: Register\nUI: Initialize\nUI: Front Panel State >> Hide", "State(s) in (\"\")"=w360) -> ("States Out"=w359:string)  [unwired: 13 in]
      }
      frame "Macro: Exit" {
        # "Exit Macro\n(This is called once, when the VI exits)"
        n127 = Unbundle By Name(w368) -> ("Core.Close Panel on Exit?"=w363:bool)
        n128 = call <vilib>:"Conditional State String__jki_lib_state_machine.vi"("Do State(s)?"=w363, "State"="UI: Front Panel State >> Close") -> ("State Out"=w362:string)  [unwired: 7 in]
        n129 = call <vilib>:"Add State(s) to Queue__jki_lib_state_machine.vi"("State(s) in (\"\")"=w362, "State(s) at Back (\"\")"="UI: Uninitialize\nData: Cleanup\nEvents: Unregister\nExit") -> ("States Out"=w366:string)  [unwired: 13 in]
        n130 = call <vilib>:"Add State(s) to Queue__jki_lib_state_machine.vi"("State(s) in Front (\"\")"=w366, "State(s) in (\"\")"=w370) -> ("States Out"=w369:string)  [unwired: 13 in]
      }
      frame "---------- Action ----------" {
        # "Template Separator\n(You can make a copy of, or modify, this frame)"
        n131 = call <vilib>:"Add State(s) to Queue__jki_lib_state_machine.vi"("State(s) in (\"\")"=w375) -> ("States Out"=w374:string)  [unwired: 14 in]
      }
      frame "Action: Periodic Work" {
        # "Your code here.\n(You can make a copy of, or modify, this frame)"
        n132 = call "Send Monitor.vi"("Message Enqueuer"=w376) -> ()  [unwired: 9 in, 2 out]
        n133 = call <vilib>:"Add State(s) to Queue__jki_lib_state_machine.vi"("State(s) in (\"\")"=w381) -> ("States Out"=w380:string)  [unwired: 14 in]
      }
      frame "Action: Connection" {
        # "Your code here.\n(You can make a copy of, or modify, this frame)"
        n134 = call "Send Connection.vi"("Message Enqueuer"=w382) -> ()  [unwired: 8 in, 3 out]
        n135 = call <vilib>:"Add State(s) to Queue__jki_lib_state_machine.vi"("State(s) in (\"\")"=w387) -> ("States Out"=w386:string)  [unwired: 14 in]
      }
      frame "Action: Disconnection" {
        # "Your code here.\n(You can make a copy of, or modify, this frame)"
        n136 = call "Send Disconnection.vi"("Message Enqueuer"=w388) -> ()  [unwired: 9 in, 2 out]
        n137 = call <vilib>:"Add State(s) to Queue__jki_lib_state_machine.vi"("State(s) in (\"\")"=w393) -> ("States Out"=w392:string)  [unwired: 14 in]
      }
      frame "---------- Listbox ----------" {
        # "Template Separator\n(You can make a copy of, or modify, this frame)"
        n138 = call <vilib>:"Add State(s) to Queue__jki_lib_state_machine.vi"("State(s) in (\"\")"=w398) -> ("States Out"=w397:string)  [unwired: 14 in]
      }
      frame "Listbox: Add Item" {
        # "Template Separator\n(You can make a copy of, or modify, this frame)"
        n139 = call "Send EditPanel.vi"("Option"=enum16{"Add", "Edit"}."Add", "Message Enqueuer"=w399) -> ()  [unwired: 8 in, 2 out]
        n140 = call <vilib>:"Add State(s) to Queue__jki_lib_state_machine.vi"("State(s) in (\"\")"=w405) -> ("States Out"=w404:string)  [unwired: 14 in]
      }
      frame "Listbox: Edit Item" {
        # "Template Separator\n(You can make a copy of, or modify, this frame)"
        n141 = call "Send EditPanel.vi"("Option"=enum16{"Add", "Edit"}."Edit", "Message Enqueuer"=w407) -> ()  [unwired: 8 in, 2 out]
        n142 = call <vilib>:"Add State(s) to Queue__jki_lib_state_machine.vi"("State(s) in (\"\")"=w412) -> ("States Out"=w411:string)  [unwired: 14 in]
      }
      frame "Listbox: Set Value" {
        # "Template Separator\n(You can make a copy of, or modify, this frame)"
        n143 = call <vilib>:"Add State(s) to Queue__jki_lib_state_machine.vi"("State(s) in (\"\")"=w417) -> ("States Out"=w416:string)  [unwired: 14 in]
      }
      frame "Listbox: Save Config" {
        # "Template Separator\n(You can make a copy of, or modify, this frame)"
        n144 = property class="PLC_Module.lvclass"(reference=w421) -> ("Acessors:Configuration"=w420:T9, "Acessors:ModuleName"=w419:string, "Acessors:ConnectConfig"=w418:T12)  [unwired: 1 in, 2 out]
        n145 = call "SaveConfigFile.vi"("ConnectConfig"=w418, "Model Name"=w419, "Configuration"=w420) -> ()  [unwired: 8 in, 1 out]
        n146 = call <vilib>:"Add State(s) to Queue__jki_lib_state_machine.vi"("State(s) in (\"\")"=w426) -> ("States Out"=w425:string)  [unwired: 14 in]
      }
      frame "Listbox: Delete Item" {
        # "Template Separator\n(You can make a copy of, or modify, this frame)"
        n147 = call "Send Delete Item.vi"("Message Enqueuer"=w427) -> ()  [unwired: 9 in, 2 out]
        n148 = call <vilib>:"Add State(s) to Queue__jki_lib_state_machine.vi"("State(s) in (\"\")"=w432) -> ("States Out"=w431:string)  [unwired: 14 in]
      }
      frame "Listbox: Edit Connect" {
        # "Template Separator\n(You can make a copy of, or modify, this frame)"
        n149 = property class="PLC_Module.lvclass"(reference=w436) -> (reference out=w435:refnum<class "PLC_Module.lvclass">, "Acessors:ConnectConfig"=w434:T12)  [unwired: 1 in, 1 out]
        n150 = call "EditConnect.vi"("ConnectConfig in"=w434) -> ("ConnectConfig out"=w433:T12)  [unwired: 10 in]
        n151 = property class="PLC_Module.lvclass"(reference=w435, "Acessors:ConnectConfig"=w433) -> ()  [unwired: 1 in, 2 out]
        n152 = call <vilib>:"Add State(s) to Queue__jki_lib_state_machine.vi"("State(s) in (\"\")"=w441) -> ("States Out"=w440:string)  [unwired: 14 in]
      }
      frame "Listbox: Duplicate Item" {
        # "Template Separator\n(You can make a copy of, or modify, this frame)"
        n153 = call "Send DuplicateItem.vi"("Message Enqueuer"=w442) -> ()  [unwired: 9 in, 2 out]
        n154 = call <vilib>:"Add State(s) to Queue__jki_lib_state_machine.vi"("State(s) in (\"\")"=w447) -> ("States Out"=w446:string)  [unwired: 14 in]
      }
    }
  }
  n155 = call-parent "Actor Core.vi"("error in"=w2, "Actor in"=w1) -> ("error out"=→"error out":errorcluster, "Actor out"=→"Actor out":refnum<class "Actor.lvclass">)  [unwired: 8 in]
